vi "作业4数字PID.vi"() -> ()   [LabVIEW 2017]
uses:
  <vilib>/addons/control/pid/pid.llb/PID (DBL).vi
  <vilib>/addons/control/pid/NI_PID_pid.lvlib
panel:
  in  "PID控制参数":cluster{"P":dbl, "I":dbl, "D":dbl}
  out "波形图表":cluster{"设备输出":dbl, "设定值":dbl}(graph)
  in  "设定值":dbl
  in  "停止":bool
  # "比例"
  # "积分"
  # "微分"
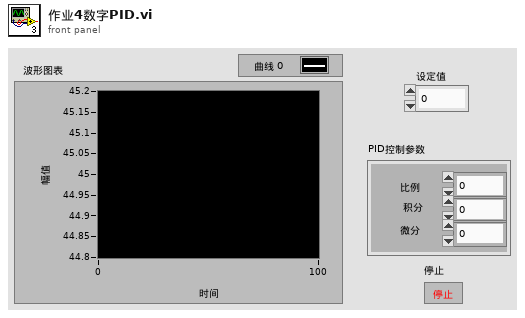
[diagram p1: front panel]
types:
  T1 = cluster{"static gain":dbl, "lag (min)":dbl, "dead cycles":dbl, "load %":dbl, "deadband":dbl, "noise level %":dbl, "initial PV":dbl, "initial PV 2":dbl}
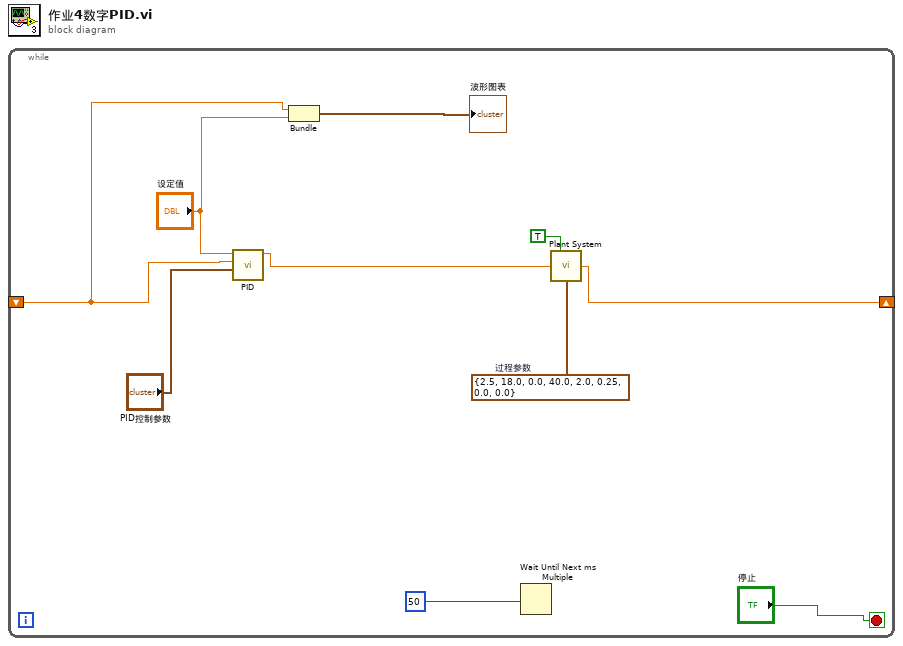
[diagram p0: block diagram]
diagram:
  n1 = while {
    shift-right: [w9] -> _
    shift-left: _ -> [w3]
    stop <- "停止" stop-if-true
    w7 = T1 {"static gain"=2.5, "lag (min)"=18.0, "dead cycles"=0.0, "load %"=40.0, "deadband"=2.0, "noise level %"=0.25, "initial PV"=0.0, "initial PV 2"=0.0}  # 过程参数
    n2 = call-poly <vilib>:"PID.vi"("PID gains"="PID控制参数", "process variable"=w3, "setpoint"="设定值") -> ("output"=w8:dbl)  [unwired: 7 in, 1 out]
    n3 = Bundle("设备输出"=w3, "设定值"="设定值") -> (→"波形图表":cluster{"设备输出":dbl, "设定值":dbl})  [unwired: 1 in]
    n4 = Wait Until Next ms Multiple(millisecond multiple=50) -> ()  [unwired: 1 out]
    n5 = call "Plant System.vi"("积分器？"=TRUE ("Integrator ?"), "设备输入"=w8, "过程参数"=w7) -> ("设备输出"=w9:dbl)  [unwired: 12 in]
  }
